vi "Node - Byte Buffer Read.vi"(8 "error in (no error)":errorcluster, 10 "Node Local Channels In":T1[](array[typedef]), 11 "Byte Buffer In":refnum<class "Byte Buffer.lvclass">) -> (0 "error out":errorcluster, 1 "Channel Data Out":dbl[](array[numeric]), 2 "Node Local Channels Out":T1[](array[typedef]), 3 "Byte Buffer Out":refnum<class "Byte Buffer.lvclass">)   [LabVIEW 2016, in "PXImc Router.lvlib"]
uses:
  PXImc Router.lvlib
  Controls/Node/Node Ch Properties.ctl
  Controls/Data Type.ctl
  <vilib>/NI Veristand/VeriStand Data/Byte Buffer/Byte Buffer.lvclass
  <vilib>/NI Veristand/VeriStand Data/Byte Buffer/Byte Buffer.lvclass/Byte Buffer.ctl
  <vilib>/NI Veristand/VeriStand Data/Byte Buffer/Byte Buffer.Read (Boolean).vi
  <vilib>/NI Veristand/VeriStand Data/Type Conversion/Type Conversion.To Double (Boolean).vi
  <vilib>/NI Veristand/VeriStand Data/Byte Buffer/Byte Buffer.Read (SGL).vi
  <vilib>/NI Veristand/VeriStand Data/Type Conversion/Type Conversion.To Double (SGL).vi
  <vilib>/NI Veristand/VeriStand Data/Byte Buffer/Byte Buffer.Read (DBL).vi
  <vilib>/NI Veristand/VeriStand Data/Byte Buffer/Byte Buffer.Read (I8).vi
  <vilib>/NI Veristand/VeriStand Data/Type Conversion/Type Conversion.To Double (I8).vi
  <vilib>/NI Veristand/VeriStand Data/Byte Buffer/Byte Buffer.Read (I16).vi
  <vilib>/NI Veristand/VeriStand Data/Type Conversion/Type Conversion.To Double (I16).vi
  <vilib>/NI Veristand/VeriStand Data/Byte Buffer/Byte Buffer.Read (I32).vi
  <vilib>/NI Veristand/VeriStand Data/Type Conversion/Type Conversion.To Double (I32).vi
  <vilib>/NI Veristand/VeriStand Data/Byte Buffer/Byte Buffer.Read (I64).vi
  <vilib>/NI Veristand/VeriStand Data/Type Conversion/Type Conversion.To Double (I64).vi
  <vilib>/NI Veristand/VeriStand Data/Byte Buffer/Byte Buffer.Read (U8).vi
  <vilib>/NI Veristand/VeriStand Data/Type Conversion/Type Conversion.To Double (U8).vi
  <vilib>/NI Veristand/VeriStand Data/Byte Buffer/Byte Buffer.Read (U16).vi
  <vilib>/NI Veristand/VeriStand Data/Type Conversion/Type Conversion.To Double (U16).vi
  <vilib>/NI Veristand/VeriStand Data/Byte Buffer/Byte Buffer.Read (U32).vi
  <vilib>/NI Veristand/VeriStand Data/Type Conversion/Type Conversion.To Double (U32).vi
  <vilib>/NI Veristand/VeriStand Data/Byte Buffer/Byte Buffer.Read (U64).vi
  <vilib>/NI Veristand/VeriStand Data/Type Conversion/Type Conversion.To Double (U64).vi
  <vilib>/NI Veristand/VeriStand Data/Byte Buffer/Byte Buffer.Read.Typed String.vi
  <vilib>/NI Veristand/VeriStand Data/Byte Buffer/Byte Buffer.Subset.Get.vi
  <vilib>/NI Veristand/VeriStand Data/Utilities/Utilities.Sizeof.Array.vi
  <vilib>/NI Veristand/VeriStand Data/Utilities/Utilities.Buffer.String.vi
  <vilib>/NI Veristand/VeriStand Data/Byte Buffer/Byte Buffer.Get Buffer Size.vi
  <vilib>/NI Veristand/VeriStand Data/Memory Management/Memory Management.MoveByteBlock.Write (String).vi
  <vilib>/NI Veristand/VeriStand Data/Byte Buffer/Byte Buffer.Get Buffer Pointer.vi
  <vilib>/NI Veristand/VeriStand Data/Utilities/Utilities.Sizeof.Scalar.vi
  <vilib>/NI Veristand/VeriStand Data/Byte Buffer/Byte Buffer.Get Byte Order.vi
  <vilib>/NI Veristand/VeriStand Data/Memory Management/Memory Management.Handle Return.vi
  <vilib>/NI Veristand/VeriStand Data/VeriStand Data.lvlib
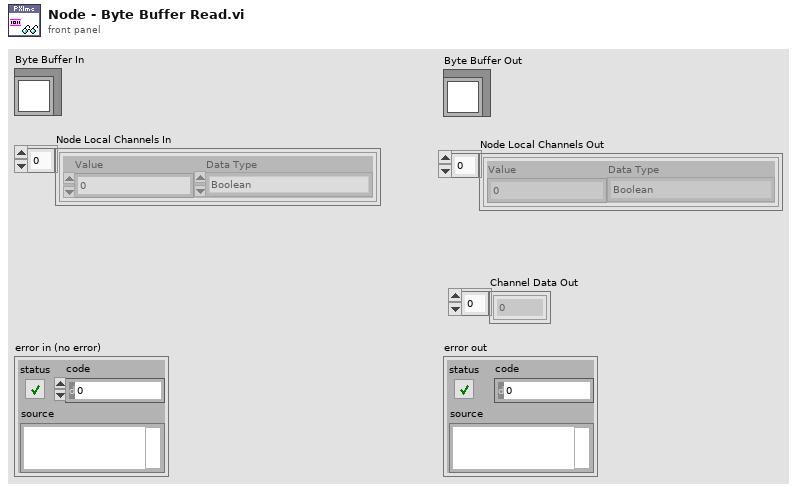
[diagram p1: front panel]
types:
  T1 = typedef "PXImc Router.lvlib/Node Ch Properties.ctl" = cluster{"Value":dbl, "Data Type":T2}
  T2 = typedef "PXImc Router.lvlib/Data Type.ctl" = enum16{"Boolean", "SGL", "DBL", "I8", "I16", "I32", "I64", "U8", "U16", "U32", "U64"}
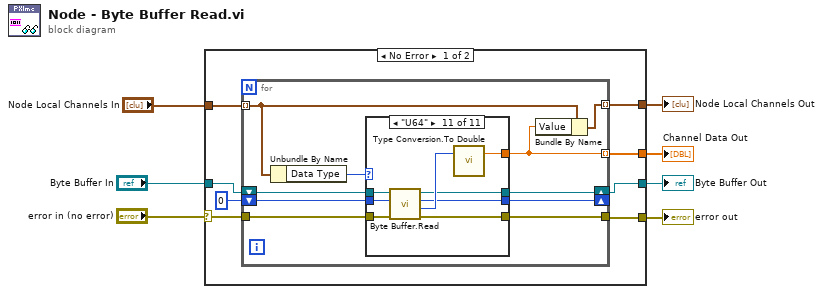
[diagram p0: block diagram]
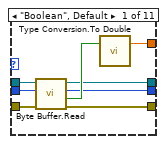
[diagram p2: hidden frame]
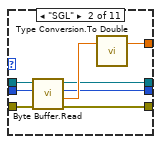
[diagram p3: hidden frame]
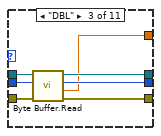
[diagram p4: hidden frame]
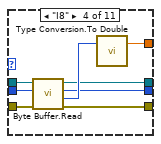
[diagram p5: hidden frame]
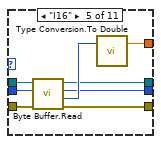
[diagram p6: hidden frame]
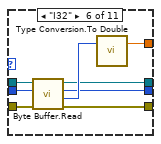
[diagram p7: hidden frame]
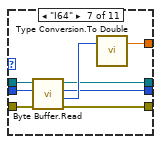
[diagram p8: hidden frame]
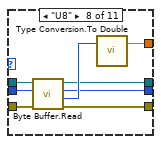
[diagram p9: hidden frame]
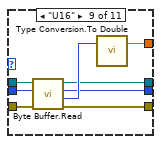
[diagram p10: hidden frame]
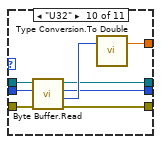
[diagram p11: hidden frame]
diagram:
  n1 = case shown="No Error" "error in (no error)" {
    selector: "error in (no error)" -> [w10 w114]
    tunnel: "Node Local Channels In" -> [w15 w113]
    tunnel: [w14 w114] -> w6
    tunnel: [w13 w115] -> w5
    tunnel: "Byte Buffer In" -> [w11 w115]
    tunnel: [w9 w113] -> w2
    tunnel: [w8 _] -> w1
    frame No Error {
      n2 = for {
        tunnel: [w20] -> w14
        shift-right: [w24] -> w13
        shift-left: w11 -> [w25]
        shift-right: [w21] -> _
        shift-left: u64 0 ("new buffer offset") -> [w22]
        tunnel: w10 -> [w23]
        tunnel: w15 -> [w18] mode=indexing
        tunnel: [w17] -> w9 mode=indexing
        tunnel: [w16] -> w8 mode=indexing
        n3 = Unbundle By Name(w18) -> ("Data Type"=w19:T2)
        n4 = case shown="\"U64\"" w19 {
          tunnel: [w32 w40 w42 w55 w63 w71 w79 w87 w95 w103 w111] -> w16
          tunnel: w25 -> [w31 w39 w48 w54 w62 w70 w78 w86 w94 w102 w110]
          tunnel: [w30 w38 w47 w53 w61 w69 w77 w85 w93 w101 w109] -> w24
          tunnel: w23 -> [w29 w37 w46 w52 w60 w68 w76 w84 w92 w100 w108]
          tunnel: w22 -> [w28 w36 w45 w51 w59 w67 w75 w83 w91 w99 w107]
          tunnel: [w27 w35 w44 w50 w58 w66 w74 w82 w90 w98 w106] -> w21
          tunnel: [w26 w34 w43 w49 w57 w65 w73 w81 w89 w97 w105] -> w20
          frame "Boolean", Default {
            n5 = call-poly <vilib>:"Byte Buffer.Read.vi"("error in (no error)"=w29, "buffer offset"=w28, "Byte Buffer in"=w31) -> ("error out"=w26:errorcluster, "value"=w33:bool, "new buffer offset"=w27:u64, "Byte Buffer out"=w30:refnum<class "Byte Buffer.lvclass">)  [unwired: 5 in]
            n6 = call-poly <vilib>:"Type Conversion.To Double.vi"("value in"=w33) -> ("value out"=w32:dbl)  [unwired: 2 in]
          }
          frame "SGL" {
            n7 = call-poly <vilib>:"Byte Buffer.Read.vi"("error in (no error)"=w37, "buffer offset"=w36, "Byte Buffer in"=w39) -> ("error out"=w34:errorcluster, "value"=w41:sgl, "new buffer offset"=w35:u64, "Byte Buffer out"=w38:refnum<class "Byte Buffer.lvclass">)  [unwired: 5 in]
            n8 = call-poly <vilib>:"Type Conversion.To Double.vi"("value in"=w41) -> ("value out"=w40:dbl)  [unwired: 2 in]
          }
          frame "DBL" {
            n9 = call-poly <vilib>:"Byte Buffer.Read.vi"("error in (no error)"=w46, "buffer offset"=w45, "Byte Buffer in"=w48) -> ("error out"=w43:errorcluster, "value"=w42:dbl, "new buffer offset"=w44:u64, "Byte Buffer out"=w47:refnum<class "Byte Buffer.lvclass">)  [unwired: 5 in]
          }
          frame "I8" {
            n10 = call-poly <vilib>:"Byte Buffer.Read.vi"("error in (no error)"=w52, "buffer offset"=w51, "Byte Buffer in"=w54) -> ("error out"=w49:errorcluster, "value"=w56:i8, "new buffer offset"=w50:u64, "Byte Buffer out"=w53:refnum<class "Byte Buffer.lvclass">)  [unwired: 5 in]
            n11 = call-poly <vilib>:"Type Conversion.To Double.vi"("value in"=w56) -> ("value out"=w55:dbl)  [unwired: 2 in]
          }
          frame "I16" {
            n12 = call-poly <vilib>:"Byte Buffer.Read.vi"("error in (no error)"=w60, "buffer offset"=w59, "Byte Buffer in"=w62) -> ("error out"=w57:errorcluster, "value"=w64:i16, "new buffer offset"=w58:u64, "Byte Buffer out"=w61:refnum<class "Byte Buffer.lvclass">)  [unwired: 5 in]
            n13 = call-poly <vilib>:"Type Conversion.To Double.vi"("value in"=w64) -> ("value out"=w63:dbl)  [unwired: 2 in]
          }
          frame "I32" {
            n14 = call-poly <vilib>:"Byte Buffer.Read.vi"("error in (no error)"=w68, "buffer offset"=w67, "Byte Buffer in"=w70) -> ("error out"=w65:errorcluster, "value"=w72:i32, "new buffer offset"=w66:u64, "Byte Buffer out"=w69:refnum<class "Byte Buffer.lvclass">)  [unwired: 5 in]
            n15 = call-poly <vilib>:"Type Conversion.To Double.vi"("value in"=w72) -> ("value out"=w71:dbl)  [unwired: 2 in]
          }
          frame "I64" {
            n16 = call-poly <vilib>:"Byte Buffer.Read.vi"("error in (no error)"=w76, "buffer offset"=w75, "Byte Buffer in"=w78) -> ("error out"=w73:errorcluster, "value"=w80:i64, "new buffer offset"=w74:u64, "Byte Buffer out"=w77:refnum<class "Byte Buffer.lvclass">)  [unwired: 5 in]
            n17 = call-poly <vilib>:"Type Conversion.To Double.vi"("value in"=w80) -> ("value out"=w79:dbl)  [unwired: 2 in]
          }
          frame "U8" {
            n18 = call-poly <vilib>:"Byte Buffer.Read.vi"("error in (no error)"=w84, "buffer offset"=w83, "Byte Buffer in"=w86) -> ("error out"=w81:errorcluster, "value"=w88:u8, "new buffer offset"=w82:u64, "Byte Buffer out"=w85:refnum<class "Byte Buffer.lvclass">)  [unwired: 5 in]
            n19 = call-poly <vilib>:"Type Conversion.To Double.vi"("value in"=w88) -> ("value out"=w87:dbl)  [unwired: 2 in]
          }
          frame "U16" {
            n20 = call-poly <vilib>:"Byte Buffer.Read.vi"("error in (no error)"=w92, "buffer offset"=w91, "Byte Buffer in"=w94) -> ("error out"=w89:errorcluster, "value"=w96:u16, "new buffer offset"=w90:u64, "Byte Buffer out"=w93:refnum<class "Byte Buffer.lvclass">)  [unwired: 5 in]
            n21 = call-poly <vilib>:"Type Conversion.To Double.vi"("value in"=w96) -> ("value out"=w95:dbl)  [unwired: 2 in]
          }
          frame "U32" {
            n22 = call-poly <vilib>:"Byte Buffer.Read.vi"("error in (no error)"=w100, "buffer offset"=w99, "Byte Buffer in"=w102) -> ("error out"=w97:errorcluster, "value"=w104:u32, "new buffer offset"=w98:u64, "Byte Buffer out"=w101:refnum<class "Byte Buffer.lvclass">)  [unwired: 5 in]
            n23 = call-poly <vilib>:"Type Conversion.To Double.vi"("value in"=w104) -> ("value out"=w103:dbl)  [unwired: 2 in]
          }
          frame "U64" {
            n24 = call-poly <vilib>:"Byte Buffer.Read.vi"("error in (no error)"=w108, "buffer offset"=w107, "Byte Buffer in"=w110) -> ("error out"=w105:errorcluster, "value"=w112:u64, "new buffer offset"=w106:u64, "Byte Buffer out"=w109:refnum<class "Byte Buffer.lvclass">)  [unwired: 5 in]
            n25 = call-poly <vilib>:"Type Conversion.To Double.vi"("value in"=w112) -> ("value out"=w111:dbl)  [unwired: 2 in]
          }
        }
        n26 = Bundle By Name(cluster=w18, "Value"=w16) -> (w17:T1)
      }
    }
    frame Error {
    }
  }
  "error out" <- w6
  "Byte Buffer Out" <- w5
  "Node Local Channels Out" <- w2
  "Channel Data Out" <- w1
